vi "Bundle Script_Named (Un)Bundler Remove Unwired.vi"(8 "error in":errorcluster, 11 "Affected Items":T1) -> (0 "error out":errorcluster, 2 "Objects":refnum<vi>[](array[refnum]))   [LabVIEW 2023]
uses:
  top/BundleMagic.ctl
panel:
  out "Unwired Indicies":i32[](array[numeric])
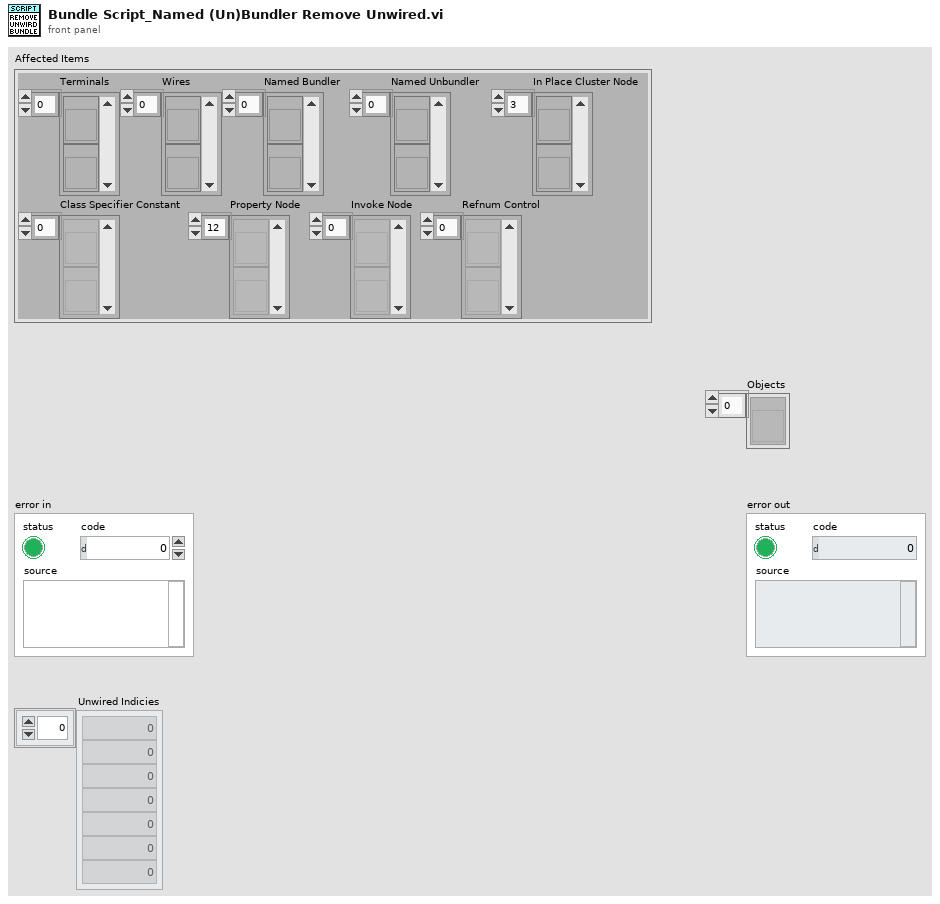
[diagram p1: front panel]
types:
  T1 = typedef "BundleMagic.ctl" = cluster{"Terminals":refnum<vi>[], "Wires":refnum<vi>[], "Named Bundler":refnum<vi>[], "Named Unbundler":refnum<vi>[], "In Place Cluster Node":refnum<vi>[], "Class Specifier Constant":refnum<vi>[], "Property Node":refnum<vi>[], "Invoke Node":refnum<vi>[], "Refnum Control":refnum<vi>[]}
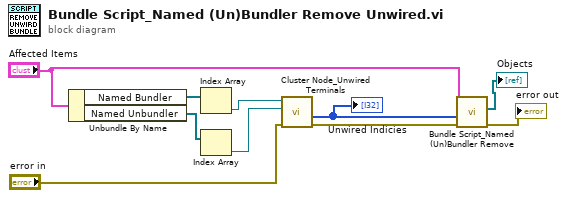
[diagram p0: block diagram]
diagram:
  n1 = Unbundle By Name("Affected Items") -> ("Named Bundler"=w7:refnum<vi>[], "Named Unbundler"=w6:refnum<vi>[])
  n2 = Index Array(array=w7) -> (element=w5:refnum<vi>)  [unwired: 1 in]
  n3 = Index Array(array=w6) -> (element=w4:refnum<vi>)  [unwired: 1 in]
  n4 = call "Cluster Node_Unwired Terminals.vi"("error in"="error in", "Named Unbundler Ref"=w4, "Named Bundler Ref"=w5) -> ("error out"=w2:errorcluster, "Unwired Indices For Removal"=w3:i32[])  [unwired: 6 in, 1 out]
  "Unwired Indicies" <- w3
  n5 = call "Bundle Script_Named (Un)Bundler Remove.vi"("error in"=w2, "Selected Item Indices"=w3, "Affected Items"="Affected Items") -> ("error out"=→"error out":errorcluster, "Objects"=→"Objects":refnum<vi>[])  [unwired: 7 in]
